vi "Get ROI length and lines.vi"(11 "Old ROI file's data in":dbl[](array[numeric])) -> (1 "Vertical":bool, 2 "Number of lines":dbl, 3 "Length":dbl)   [LabVIEW 2017]
panel:
  # "The longest dimension is output as \"Length\""
  # "The shortest dimension is output as \"Number of lines\""
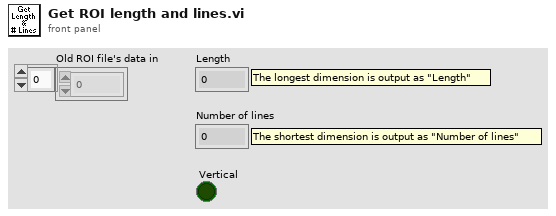
[diagram p1: front panel]
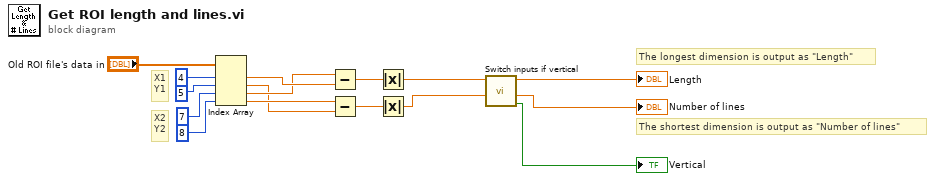
[diagram p0: block diagram]
diagram:
  # "The shortest dimension is output as \"Number of lines\""
  # "The longest dimension is output as \"Length\""
  # "X2\nY2"
  # "X1\nY1"
  n1 = Index Array(array="Old ROI file's data in", index #1=4 ("index"), index #2=5 ("index"), index #3=7 ("index"), index #4=8 ("index")) -> (element #1=w11:dbl, element #2=w8:dbl, element #3=w9:dbl, element #4=w10:dbl)
  n2 = Subtract(x=w9, y=w11) -> (x-y=w12:dbl)
  n3 = Subtract(x=w10, y=w8) -> (x-y=w13:dbl)
  n4 = Absolute Value(x=w12) -> (abs(x)=w14:dbl)
  n5 = Absolute Value(x=w13) -> (abs(x)=w15:dbl)
  n6 = call "Switch inputs if vertical.vi"("Y length"=w15, "X length"=w14) -> ("Vertical"=→"Vertical":bool, "Number of lines"=→"Number of lines":dbl, "Length"=→"Length":dbl)  [unwired: 7 in]
